vi "FTW-JSON-Destroy.vi"(0 "JSON Object":refnum<data-value>, 11 "error in":errorcluster) -> (15 "error out":errorcluster)   [LabVIEW 2015]
uses:
  core/FTW-JSON-Core-Structure.ctl
  error/FTW-ERR-ThrowError.vi
  error/FTW-ERR-CallChain.vi
  string/FTW-STR-ReplaceWhitespace.vi
  string/FTW-STR-Array-Delimit.vi
  error/FTW-ERR-Clear.vi
  regex/FTW-Regex-ReplaceAll.vi
panel:
  # "Inputs"
  # "Outputs"
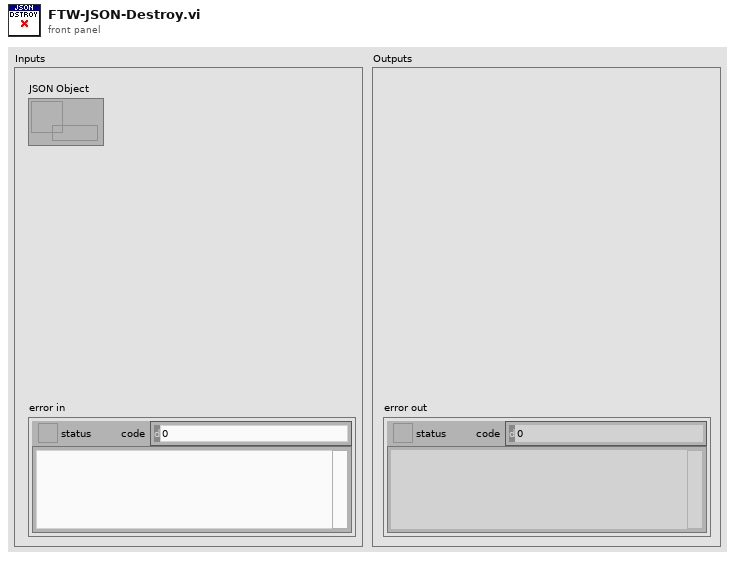
[diagram p1: front panel]
types:
  T1 = typedef "FTW-JSON-Core-Structure.ctl" = cluster{"JSON Object":i64, "Encoding Flags":i64, "Decoding Flags":i64}
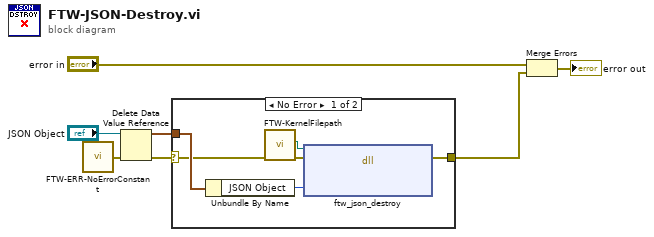
[diagram p0: block diagram]
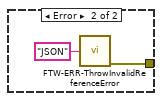
[diagram p2: hidden frame]
diagram:
  n1 = call "FTW-ERR-NoErrorConstant.vi"() -> ("no error"=w1:errorcluster)
  n2 = Delete Data Value Reference(data value reference="JSON Object", error in=w1) -> (data value=w3:T1, error out=w2:errorcluster)
  n3 = case shown="No Error" w2 {
    selector: w2 -> [w10 _]
    tunnel: [w13 w15] -> w6
    tunnel: w3 -> [w12 _]
    frame No Error {
      n4 = Unbundle By Name(w12) -> ("JSON Object"=w11:i64)
      n5 = call "FTW-KernelFilepath.vi"("error in"=w10) -> ("error out"=w9:errorcluster, "Library Filepath"=w8:path)  [unwired: 8 in, 1 out]
      n6 = dll-call lib="?" fn="ftw_json_destroy"(path in=w8, error in=w9, "JSON Object Pointer"=w11) -> (error out=w13:errorcluster)  [unwired: 3 in, 1 out]
    }
    frame Error {
      n7 = call "FTW-ERR-ThrowInvalidReferenceError.vi"("Reference Type"="JSON") -> ("error out"=w15:errorcluster)  [unwired: 14 in]
    }
  }
  n8 = Merge Errors("error in", w6) -> (→"error out":errorcluster)
